vi "Untitled 1bbbb.vi"() -> ()   [LabVIEW 2019]
uses:
  <vilib>/MakerHub/LINX/Public/Peripherals/Digital/Digital Read 1 Chan.vi
  <vilib>/MakerHub/LINX/Public/Peripherals/Digital/Digital Write 1 Chan.vi
  <vilib>/MakerHub/LINX/Public/Peripherals/Digital/Digital Read N Chans.vi
  <vilib>/MakerHub/LINX/Public/Peripherals/Digital/Digital Write N Chans.vi
  <vilib>/MakerHub/LINX/Private/Local IO/LinxDigitalRead.vi
  <vilib>/MakerHub/LINX/Public/Utilities/Check Channel.vi
  <vilib>/MakerHub/LINX/Private/Local IO/LinxDigitalWrite.vi
  <vilib>/MakerHub/LINX/Public/Utilities/Open Serial.vi
  <vilib>/MakerHub/LINX/Private/Utilties/Generate Error.vi
  <vilib>/MakerHub/LINX/LMH-LINX.lvlib
panel:
  in  "Serial Port":refnum<visa-resource-name>="N/A"
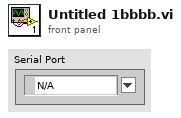
[diagram p1: front panel]
types:
  T1 = typedef "LMH-LINX.lvlib/LINX Ref.ctl" = cluster{"IO":T2, "Interface":T3, "LINX Device Config":T4}
  T2 = typedef "LMH-LINX.lvlib/Platform.ctl" = enum16{"Remote", "Local"}
  T3 = typedef "LMH-LINX.lvlib/Interface.ctl" = enum16{"Serial", "TCP"}
  T4 = typedef "LMH-LINX.lvlib/Device.lvlib/LINX Device Config.ctl" = cluster{"Interface":T3, "COM Port":refnum<visa-resource-name>, "TCP Configuration":T5, "Device Family":u8, "Device ID":u8, "Device Name":string, "TCP Ref":refnum<k5>, "Channels":T6}
  T5 = typedef "LMH-LINX.lvlib/Device.lvlib/TCP Config.ctl" = cluster{"IP Address":string, "Port":u16}
  T6 = typedef "LMH-LINX.lvlib/Channels.ctl" = cluster{"DI":u8[], "DO":u8[], "AI":u8[], "AO":u8[], "PWM":u8[], "QE":u8[], "UART":u8[], "I2C 2":u8[], "SPI":u8[], "CAN":u8[], "Servo":u8[], "AI Ref (V)":dbl, "AI Resolution (Bits)":u8, "AO Ref (V)":dbl, "AO Resolution (Bits)":u8}
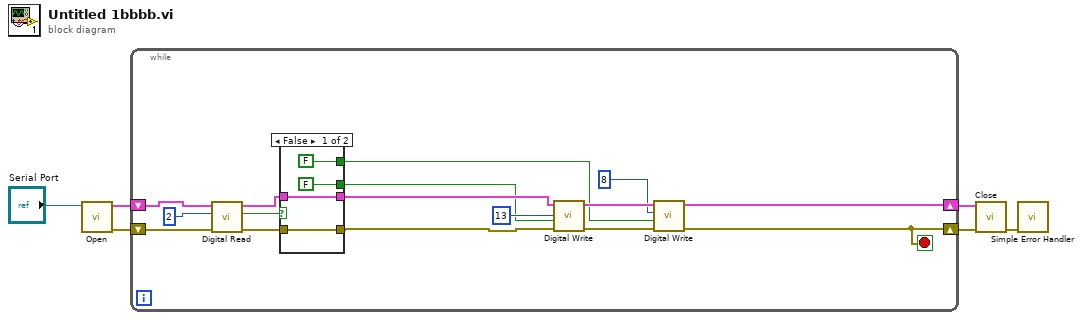
[diagram p0: block diagram]
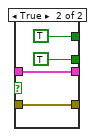
[diagram p2: hidden frame]
diagram:
  n1 = call-poly <vilib>:"Open.vi"("Serial Port"="Serial Port") -> ("Error Out"=w2:errorcluster, "LINX Resource"=w4:T1)  [unwired: 8 in, 1 out]
  n2 = while {
    shift-right: [w8] -> w1
    shift-left: w4 -> [w22]
    shift-right: [w7] -> w3
    shift-left: w2 -> [w21]
    stop <- w7 stop-if-true
    n3 = call-poly <vilib>:"Digital Read.vi"("Error In"=w21, "DI Channel"=u8 2, "LINX Resource"=w22) -> ("Error Out"=w18:errorcluster, "DI Value"=w19:bool, "LINX Resource"=w17:T1)  [unwired: 6 in]
    n4 = case shown="False" w19 {
      tunnel: [w25 w30] -> w11
      tunnel: w18 -> [w25 w30]
      tunnel: [w26 w29] -> w12
      tunnel: w17 -> [w26 w29]
      tunnel: [FALSE TRUE] -> w10
      tunnel: [FALSE TRUE] -> w9
      frame False {
      }
      frame True {
      }
    }
    n5 = call-poly <vilib>:"Digital Write.vi"("Error In"=w11, "Output Value"=w10, "DO Channel"=u8 13, "LINX Resource"=w12) -> ("Error Out"=w15:errorcluster, "LINX Resource"=w16:T1)  [unwired: 6 in]
    n6 = call-poly <vilib>:"Digital Write.vi"("Error In"=w15, "Output Value"=w9, "DO Channel"=u8 8, "LINX Resource"=w16) -> ("Error Out"=w7:errorcluster, "LINX Resource"=w8:T1)  [unwired: 6 in]
  }
  n7 = call <vilib>:"Close.vi"("Error In"=w3, "LINX Resource"=w1) -> ("Error Out"=w5:errorcluster)  [unwired: 9 in]
  n8 = call <vilib>:"Simple Error Handler.vi"("error in (no error)"=w5) -> ()  [unwired: 4 in, 5 out]
